vi "Init Loop Data.vi"(7 "UI Refs":T1, 8 "error in (no error)":errorcluster, 9 "Destinations Ref":refnum<k24>, 10 "Sources Ref":refnum<k24>, 11 "SDF Path":path) -> (0 "error out":errorcluster, 3 "Loop Data":T2)   [LabVIEW 2016, in "System Mapping Tool.lvlib"]
uses:
  System Mapping Tool.lvlib
  TypeDefs/Loop Data.ctl
  TypeDefs/UI Refs.ctl
  NationalInstruments.VeriStand.SystemDefinitionAPI
  NationalInstruments.VeriStand.SystemStorageUI
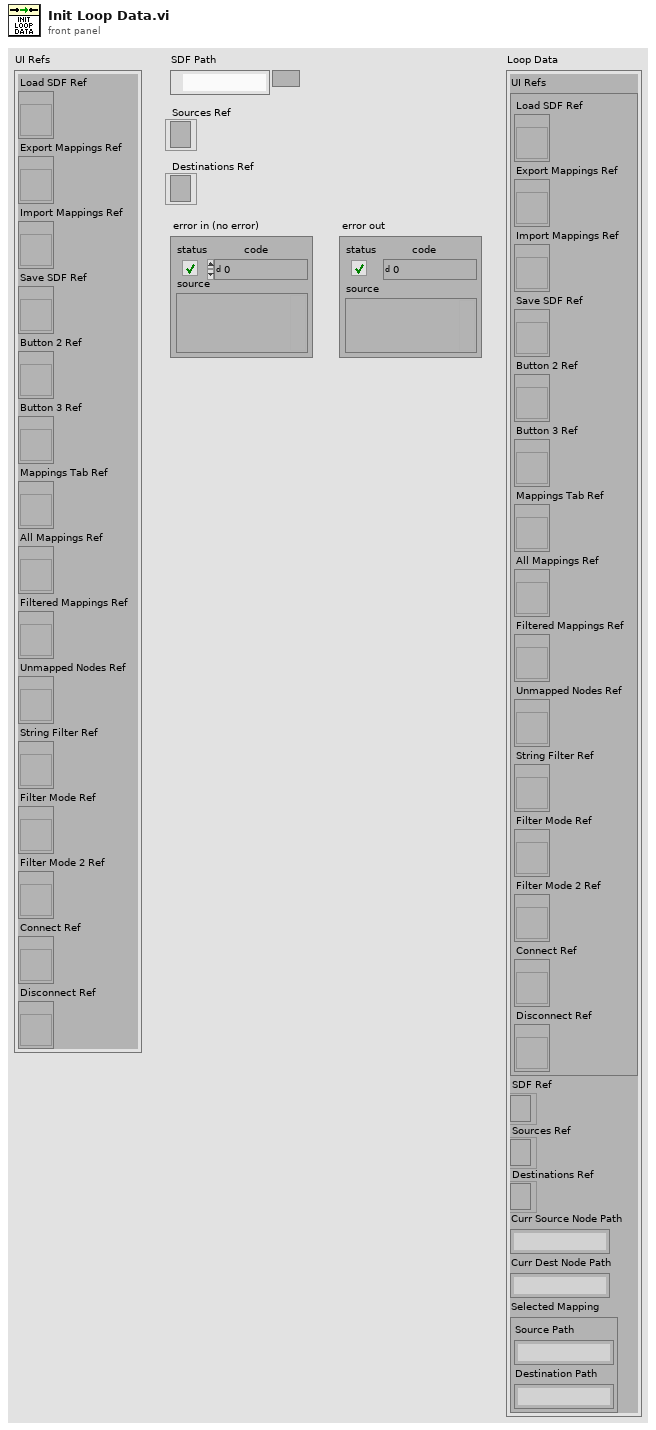
[diagram p1: front panel]
types:
  T1 = typedef "System Mapping Tool.lvlib/UI Refs.ctl" = cluster{"Load SDF Ref":refnum<vi>, "Export Mappings Ref":refnum<vi>, "Import Mappings Ref":refnum<vi>, "Save SDF Ref":refnum<vi>, "Button 2 Ref":refnum<vi>, "Button 3 Ref":refnum<vi>, "Mappings Tab Ref":refnum<vi>, "All Mappings Ref":refnum<vi>, "Filtered Mappings Ref":refnum<vi>, "Unmapped Nodes Ref":refnum<vi>, "String Filter Ref":refnum<vi>, "Filter Mode Ref":refnum<vi>, "Filter Mode 2 Ref":refnum<vi>, "Connect Ref":refnum<vi>, "Disconnect Ref":refnum<vi>}
  T2 = typedef "System Mapping Tool.lvlib/Loop Data.ctl" = cluster{"UI Refs":T1, "SDF Ref":refnum<k24>, "Sources Ref":refnum<k24>, "Destinations Ref":refnum<k24>, "Curr Source Node Path":string, "Curr Dest Node Path":string, "Selected Mapping":cluster{"Source Path":string, "Destination Path":string}}
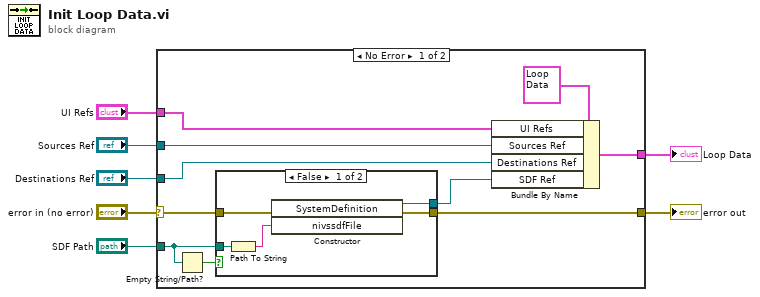
[diagram p0: block diagram]
diagram:
  n1 = case shown="No Error" "error in (no error)" {
    selector: "error in (no error)" -> [w17 w24]
    tunnel: [w11 w24] -> w6
    tunnel: "SDF Path" -> [w9 _]
    tunnel: "Destinations Ref" -> [w14 _]
    tunnel: "Sources Ref" -> [w13 _]
    tunnel: "UI Refs" -> [w12 _]
    tunnel: [w10 _] -> w1
    frame No Error {
      n2 = Empty String/Path?(string/path=w9) -> (empty?=w8:bool)
      n3 = case shown="False" w8 {
        tunnel: w17 -> [w22 w23]
        tunnel: w9 -> [w21 _]
        tunnel: [w19 _] -> w15
        tunnel: [w18 w23] -> w11
        frame False {
          n4 = Path To String(path=w21) -> (string=w20:string)
          n5 = constructor class="SystemDefinition"(error in=w22, "nivssdfFile"=w20) -> (reference out=w19:refnum<k24>, error out=w18:errorcluster)  [unwired: 2 in, 2 out]
        }
        frame True {
        }
      }
      n6 = Bundle By Name(cluster=T2 {"UI Refs"={"Load SDF Ref"=refnum, "Export Mappings Ref"=refnum, "Import Mappings Ref"=refnum, "Save SDF Ref"=refnum, "Button 2 Ref"=refnum, "Button 3 Ref"=refnum, "Mappings Tab Ref"=refnum, "All Mappings Ref"=refnum, "Filtered Mappings Ref"=refnum, "Unmapped Nodes Ref"=refnum, "String Filter Ref"=refnum, "Filter Mode Ref"=refnum, "Filter Mode 2 Ref"=refnum, "Connect Ref"=refnum, "Disconnect Ref"=refnum}, "SDF Ref"=refnum, "Sources Ref"=refnum, "Destinations Ref"=refnum, "Curr Source Node Path"="", "Curr Dest Node Path"="", "Selected Mapping"={"Source Path"="", "Destination Path"=""}} ("Loop Data"), "UI Refs"=w12, "Sources Ref"=w13, "Destinations Ref"=w14, "SDF Ref"=w15) -> (w10:T2)
    }
    frame Error {
    }
  }
  "Loop Data" <- w1
  "error out" <- w6
